vi "Plot_FFID_Calibs.vi"() -> ()   [LabVIEW 2016]
panel:
  out "Calib 2":cluster{dbl[], dbl[]}[](graph)
  out "Zero":cluster{dbl[], dbl[]}[](graph)
  out "Calib 1":cluster{dbl[], dbl[]}[](graph)
  in  "History (days)":i32=5 min=0
  out "Calib 3":cluster{dbl[], dbl[]}[](graph)
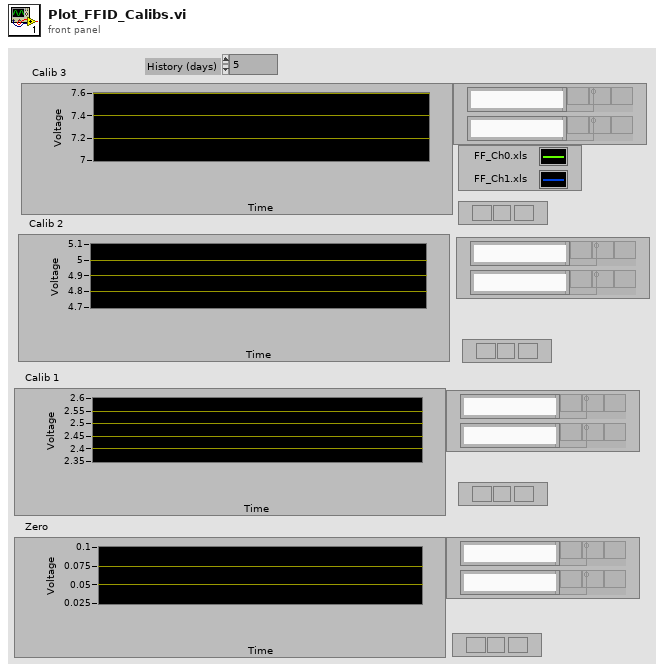
[diagram p1: front panel]
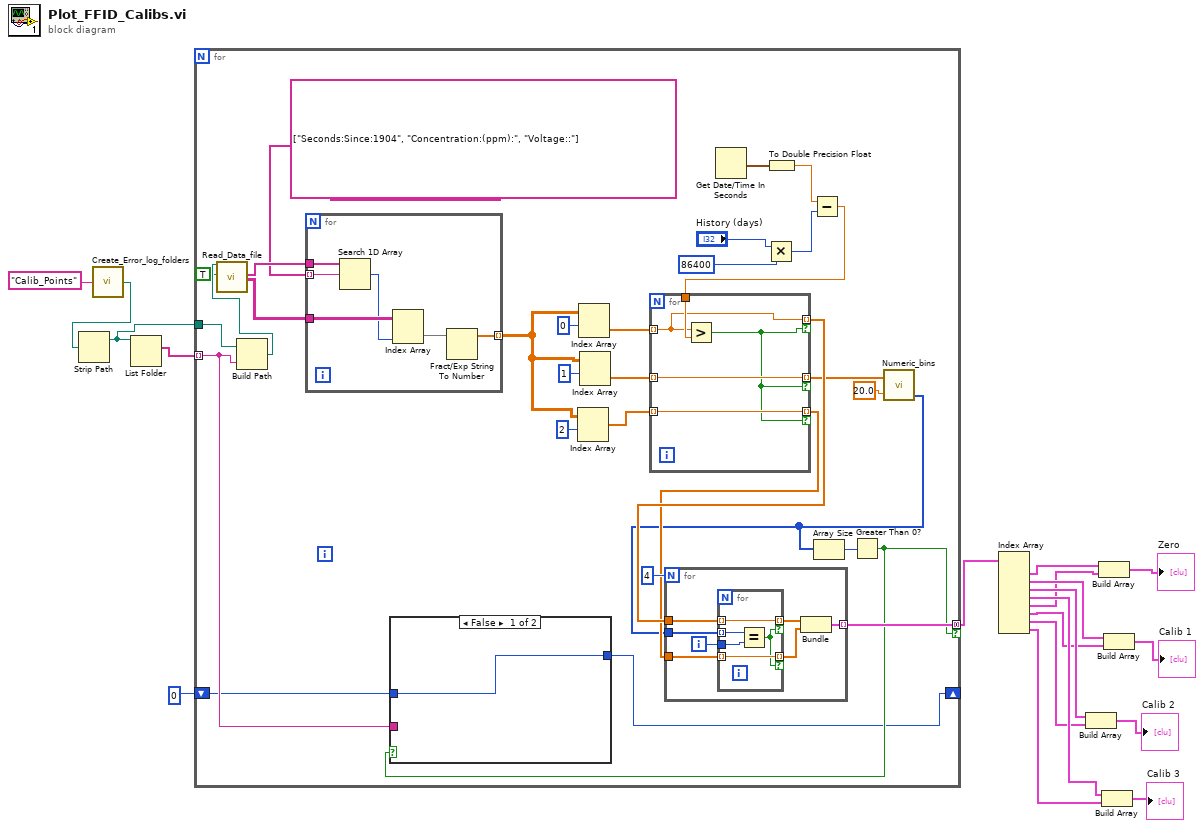
[diagram p0: block diagram]
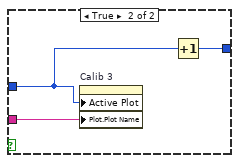
[diagram p2: hidden frame]
diagram:
  n1 = call "Create_Error_log_folders.vi"("Log Folder"="Calib_Points") -> ("Server copy Location"=w16:path)  [unwired: 2 in, 2 out]
  n2 = Strip Path(path=w16) -> (stripped path=w17:path)  [unwired: 1 out]
  n3 = List Folder(path=w17) -> (filenames=w11:string[])  [unwired: 3 in, 3 out]
  n4 = for {
    tunnel: w17 -> [w45]
    tunnel: w11 -> [w22] mode=indexing
    tunnel: [w26] -> w15 mode=concatenating if=w23
    shift-right: [w20] -> _
    shift-left: 0 -> [w21]
    n5 = Build Path(base path=w45, name or relative path=w22) -> (appended path=w44:path)
    n6 = call "Read_Data_file.vi"("Results file"=w44, "Delete First Rows?"=TRUE) -> ("Ch names Out"=w49:string[], "Channel Values Out"=w47:string[][])  [unwired: 7 in, 9 out]
    n7 = for {
      tunnel: w49 -> [w76]
      tunnel: string[] ["Seconds:Since:1904", "Concentration:(ppm):", "Voltage::"] ("Ch names Out") -> [w75] mode=indexing
      tunnel: w47 -> [w74]
      tunnel: [w71] -> w41 mode=indexing
      n8 = Search 1D Array(1D array=w76, element=w75) -> (index of element=w72:i32)  [unwired: 1 in]
      n9 = Index Array(array=w74, index (col)=w72) -> (element=w73:string[])  [unwired: 1 in]
      n10 = Fract/Exp String To Number(string=w73) -> (number=w71:dbl[])  [unwired: 3 in, 1 out]
    }
    n11 = Index Array(array=w41, index (row)=2) -> (element=w28:dbl[])  [unwired: 1 in]
    n12 = Index Array(array=w41, index (row)=0) -> (element=w32:dbl[])  [unwired: 1 in]
    n13 = Index Array(array=w41, index (row)=1) -> (element=w29:dbl[])  [unwired: 1 in]
    n14 = Get Date/Time In Seconds() -> (seconds since 1Jan1904=w38:timestamp)
    n15 = Multiply(x="History (days)", y=86400) -> (x*y=w34:i32)
    n16 = To Double Precision Float(number=w38) -> (double precision float=w35:dbl)
    n17 = Subtract(x=w35, y=w34) -> (x-y=w33:dbl)
    n18 = for {
      tunnel: w32 -> [w57] mode=indexing
      tunnel: w33 -> [w58]
      tunnel: [w57] -> w31 mode=indexing if=w54
      tunnel: [w56] -> w30 mode=indexing if=w54
      tunnel: w29 -> [w56] mode=indexing
      tunnel: [w55] -> w27 mode=indexing if=w54
      tunnel: w28 -> [w55] mode=indexing
      n19 = Greater?(x=w57, y=w58) -> (0:w54:bool)
    }
    n20 = call "Numeric_bins.vi"("Values"=w30, "Tolerance"=20.0) -> ("Bin Index"=w25:i32[])  [unwired: 2 out]
    n21 = for {
      N: 4 -> [_]
      tunnel: w25 -> [w65]
      tunnel: w31 -> [w62]
      tunnel: w27 -> [w61]
      tunnel: [w59] -> w26 mode=indexing
      i -> [w60]
      n22 = for {
        tunnel: w60 -> [w70]
        tunnel: w65 -> [w69] mode=indexing
        tunnel: [w68] -> w64 mode=indexing if=w66
        tunnel: w61 -> [w68] mode=indexing
        tunnel: [w67] -> w63 mode=indexing if=w66
        tunnel: w62 -> [w67] mode=indexing
        n23 = Equal?(x=w69, y=w70) -> (x = y?=w66:bool)
      }
      n24 = Bundle(w63, w64) -> (w59:cluster{dbl[], dbl[]})  [unwired: 1 in]
    }
    n25 = Array Size(array=w25) -> (size(s)=w24:i32)
    n26 = Greater Than 0?(x=w24) -> (x > 0?=w23:bool)
    n27 = case shown="False" w23 {
      tunnel: w22 -> [_ w53]
      tunnel: w21 -> [w50 w52]
      tunnel: [w50 w51] -> w20
      frame False {
      }
      frame True {
        n28 = property on="Calib 3" class="XYGraph (strict)"("Active Plot"=w52, "Plot.Plot Name"=w53) -> ()  [unwired: 2 in, 2 out]
        n29 = Increment(x=w52) -> (x+1=w51:i32)
      }
    }
  }
  n30 = Index Array(array=w15) -> (element #1=w14:cluster{dbl[], dbl[]}, element #2=w13:cluster{dbl[], dbl[]}, element #3=w7:cluster{dbl[], dbl[]}, element #4=w6:cluster{dbl[], dbl[]}, element #5=w5:cluster{dbl[], dbl[]}, element #6=w4:cluster{dbl[], dbl[]}, element #7=w3:cluster{dbl[], dbl[]}, element #8=w2:cluster{dbl[], dbl[]})  [unwired: 8 in]
  n31 = Build Array(w7, w3) -> (→"Calib 2":cluster{dbl[], dbl[]}[])
  n32 = Build Array(w14, w5) -> (→"Zero":cluster{dbl[], dbl[]}[])
  n33 = Build Array(w6, w2) -> (→"Calib 3":cluster{dbl[], dbl[]}[])
  n34 = Build Array(w13, w4) -> (→"Calib 1":cluster{dbl[], dbl[]}[])
